vi "Set Progression.vi"(8 "error in (no error)":errorcluster, 9 "Maximum Value (100)":u64=100, 10 "Current Value":u64, 11 "Window Handle":refnum<k24>) -> (0 "error out":errorcluster, 3 "Window Handle out":refnum<k24>)   [LabVIEW 2015, in "Simple Progress Bar.lvlib"]
uses:
  Simple Progress Bar.lvlib
  C:/Program Files (x86)/National Instruments/LabVIEW 2015/vi.lib/TaskbarProgressAPI/Windows7Taskbar.dll
  Program Files (x86)/National Instruments/LabVIEW 2015/vi.lib/TaskbarProgressAPI/Windows7Taskbar.dll
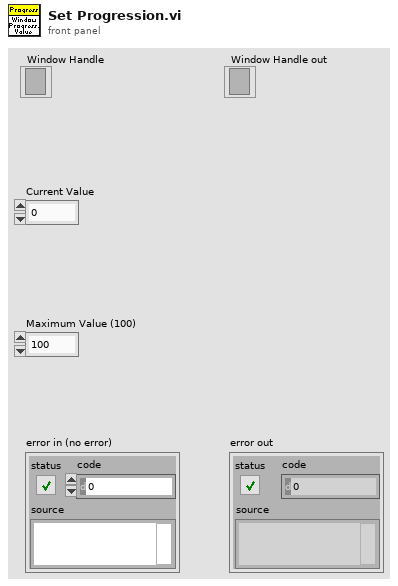
[diagram p1: front panel]
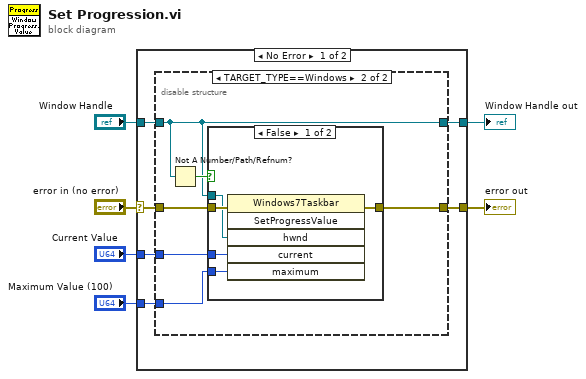
[diagram p0: block diagram]
diagram:
  n1 = case shown="No Error" "error in (no error)" {
    selector: "error in (no error)" -> [w11 w27]
    tunnel: "Window Handle" -> [w12 _]
    tunnel: [w10 w27] -> w5
    tunnel: [w9 _] -> w4
    tunnel: "Current Value" -> [w8 _]
    tunnel: "Maximum Value (100)" -> [w7 _]
    frame No Error {
      n2 = disable-structure shown="TARGET_TYPE==Windows" {
        disable-tunnel: w12 -> [w13 w17]
        disable-tunnel: w11 -> [w14 w20]
        disable-tunnel: [w14 w19] -> w10
        disable-tunnel: [w13 w17] -> w9
        disable-tunnel: w8 -> [_ w16]
        disable-tunnel: w7 -> [_ w15]
        frame condition #0 {
          # "#ToError"
        }
        frame condition #1 (active) {
          n3 = Not A Number/Path/Refnum?(number/path/refnum=w17) -> (NaN/Path/Refnum?=w18:bool)
          n4 = case shown="False" w18 {
            tunnel: w20 -> [w25 w26]
            tunnel: [w24 w26] -> w19
            tunnel: w17 -> [w23 _]
            tunnel: w16 -> [w22 _]
            tunnel: w15 -> [w21 _]
            frame False {
              n5 = invoke class="Windows7Taskbar" method="SetProgressValue"(error in=w25, "hwnd"=w23, "current"=w22, "maximum"=w21) -> (error out=w24:errorcluster)  [unwired: 2 in, 5 out]
            }
            frame True {
            }
          }
        }
      }
    }
    frame Error {
    }
  }
  "error out" <- w5
  "Window Handle out" <- w4
